vi "Get Index Directory Path.vi"(8 "error in (no error)":errorcluster) -> (0 "error out":errorcluster, 3 "Index Directory":path)   [LabVIEW 2020, in "Utilities.lvlib"]
doc: "Generates the default configuration path. \nWhen called from the development environement, the default config path is the /Config relative to the project path.\nWhen called from a built exe the default config path is at C:\\Users\\<username>\\AppData\\Local\\<CompanyName>\\<ProductName> where company name and product name are the ones configured in the build specification.\nOn Linux the default config directory is \\home\\lvuser\\natinst\\bin\\config."
uses:
  Utilities.lvlib
  <vilib>/Utility/sysdir.llb/Get System Directory.vi
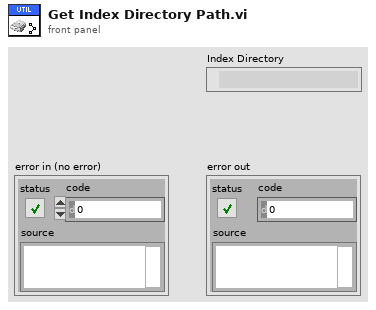
[diagram p1: front panel]
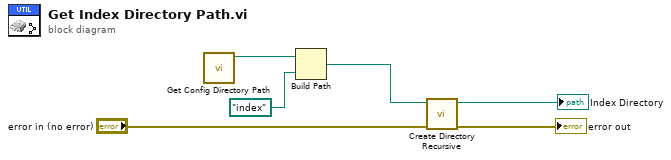
[diagram p0: block diagram]
diagram:
  n1 = call "Get Config Directory Path.vi"() -> ("Config Directory Path"=w3:path)  [unwired: 11 in]
  n2 = Build Path(base path=w3, name or relative path=path "index") -> (appended path=w2:path)
  n3 = call <vilib>:"Create Directory Recursive.vi"("error in (no error)"="error in (no error)", "directory"=w2) -> ("error out"=→"error out":errorcluster, "directory copy"=→"Index Directory":path)  [unwired: 3 in, 1 out]
